vi "Save Index to File.vi"(8 "error in (no error)":errorcluster, 10 "Project or Class Path":path, 11 "Bufferend Test Finder in":refnum<class "Indexing Test Finder.lvclass">) -> (0 "error out":errorcluster, 3 "Bufferend Test Finder out":refnum<class "Indexing Test Finder.lvclass">)   [LabVIEW 2020, in "Indexing Test Finder.lvclass"]
uses:
  Indexing Test Finder.lvclass
  Indexing Test Finder.lvclass/Indexing Test Finder.ctl
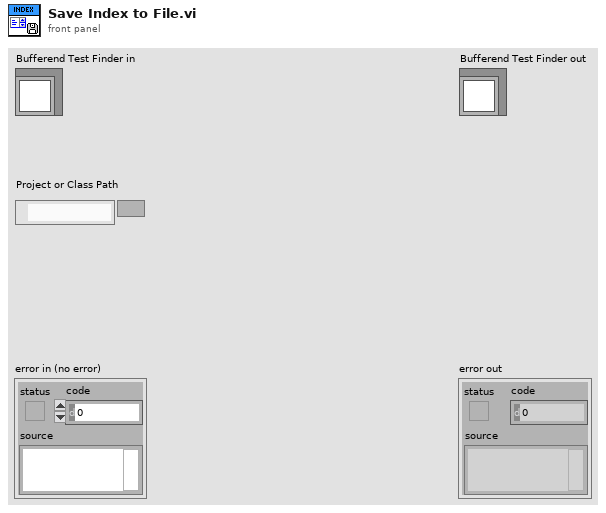
[diagram p1: front panel]
types:
  T1 = enum16{"open", "replace", "create", "open or create", "replace or create", "replace or create with confirmation"}
  T2 = typedef "Indexing Test Finder.lvclass/Index Item.ctl" = cluster{"Dynamic Methods":map{string, path}, "Static Methods":map{string, path}, "Signature":string}
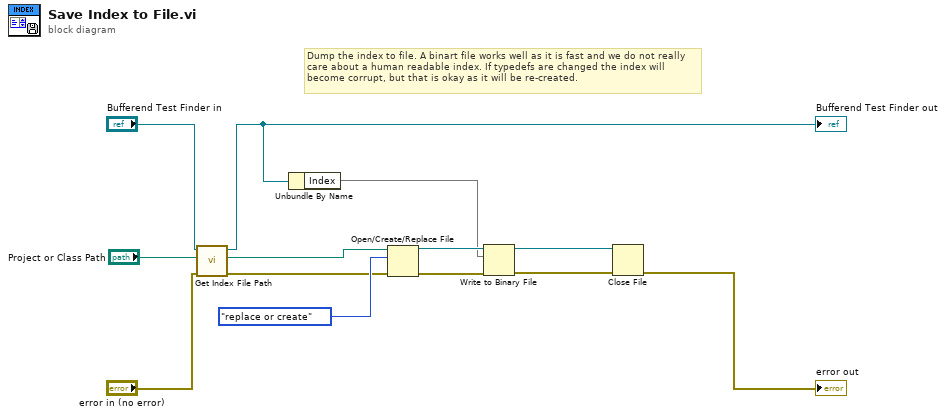
[diagram p0: block diagram]
diagram:
  # "Dump the index to file. A binart file works well as it is fast and we do not really care about a human readable index. If typedefs are changed the index will become corrupt, but that is okay as it will be re-created."
  n1 = call "Get Index File Path.vi"("error in (no error)"="error in (no error)", "Project or Class Path"="Project or Class Path", "Indexing Test Finder in"="Bufferend Test Finder in") -> ("error out"=w2:errorcluster, "Index File Path"=w3:path, "Indexing Test Finder out"=w5:refnum<class "Indexing Test Finder.lvclass">)  [unwired: 6 in]
  "Bufferend Test Finder out" <- w5
  n2 = Unbundle By Name(w5) -> ("Index"=w7:map{path, T2})
  n3 = Open/Create/Replace File(file path (use dialog)=w3, error in=w2, operation (0:open)=T1."replace or create") -> (refnum out=w12:refnum<file>, error out=w11:errorcluster)  [unwired: 3 in, 1 out]
  n4 = Write to Binary File(file (use dialog)=w12, data=w7, error in=w11) -> (refnum out=w8:refnum<file>, error out=w10:errorcluster)  [unwired: 3 in, 1 out]
  n5 = Close File(refnum=w8, error in=w10) -> (error out=→"error out":errorcluster)  [unwired: 1 out]
